vi "oct_image.vi"(11 "Sample":cluster{"img":u8[][]}={"img"=[[0, 0], [0, 0]]}) -> ()   [LabVIEW 2024]
uses:
  <vilib>/RTI DDS Toolkit/Types/RTI DDS Advanced Writer Configuration.ctl
  <vilib>/RTI DDS Toolkit/Library/LVDDS_library.lvlib
panel:
  in  "Sample Type":cluster{"img":u8[][]}={"img"=[[0, 0], [0, 0]]}
  in  "Advanced Writer Configuration":T1={"typeName"="octa_ros::msg::dds_::img_", "keyName"="", "domainParticipantQoSProfile"="", "dataWriterQoSProfile"="", "forceArrayMapping?"=FALSE, "forceUnboundedString?"=FALSE}
  in  "error in (no error)":errorcluster
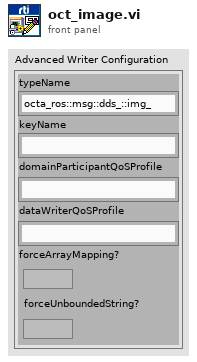
[diagram p1: front panel]
types:
  T1 = typedef "LVDDS_library.lvlib/RTI DDS Advanced Writer Configuration.ctl" = cluster{"typeName":string, "keyName":string, "domainParticipantQoSProfile":string, "dataWriterQoSProfile":string, "forceArrayMapping?":bool, "forceUnboundedString?":bool}
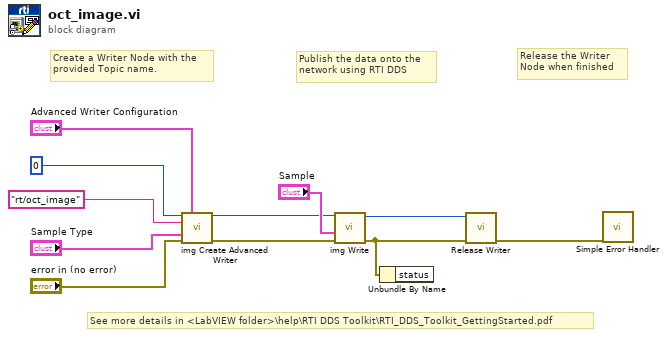
[diagram p0: block diagram]
diagram:
  # "See more details in <LabVIEW folder>\\help\\RTI DDS Toolkit\\RTI_DDS_Toolkit_GettingStarted.pdf"
  # "Release the Writer\nNode when finished"
  # "Publish the data onto the \nnetwork using RTI DDS"
  # "Create a Writer Node with the \nprovided Topic name."
  n1 = call "img Create Advanced Writer.vi"("Domain Id"=u32 0, "Advanced Writer Configuration"="Advanced Writer Configuration", "Topic Name"="rt/oct_image", "MyComplexType type"="Sample Type", "error in (no error)"="error in (no error)") -> ("DDS Object Ref"=w2:u64, "error out"=w3:errorcluster)  [unwired: 9 in]
  n2 = call "img Write.vi"("error in (no error)"=w3, "MyComplexType"="Sample", "DDS Object Ref in"=w2) -> ("error out"=w4:errorcluster, "DDS Object Ref out"=w1:u64)  [unwired: 7 in]
  n3 = Unbundle By Name(w4) -> ()  [unwired: 1 out]
  n4 = call <vilib>:"Release Writer.vi"("error in (no error)"=w4, "DDS Object Ref"=w1) -> ("error out"=w11:errorcluster)  [unwired: 9 in]
  n5 = call <vilib>:"Simple Error Handler.vi"("error in (no error)"=w11) -> ()  [unwired: 4 in, 5 out]
